vi "Get DBL.vi"(8 "error in (no error)":errorcluster, 9 "Data Type (default value)":dbl=nan, 10 "Offset":i32, 11 "JSON":string) -> (0 "error out":errorcluster, 1 "Number":dbl format="%.2f", 2 "Offset past match":i32)   [LabVIEW 2024, in "JSONtext.lvlib"]
uses:
  JSONtext.lvlib
  String Subset.vi
  Advance past Number.vi
  Parsing Error in converting to LabVIEW type.vi
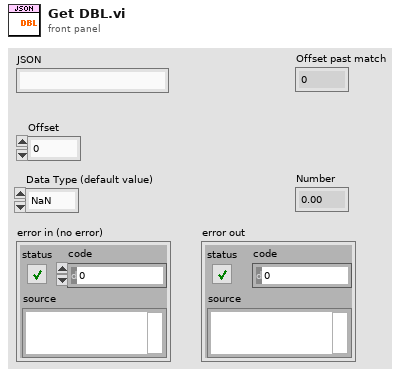
[diagram p1: front panel]
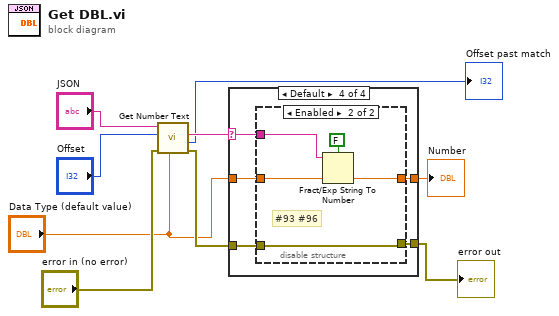
[diagram p0: block diagram]
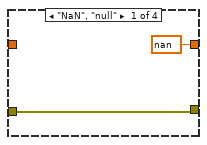
[diagram p2: hidden frame]
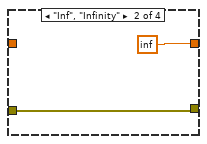
[diagram p3: hidden frame]
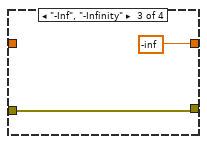
[diagram p4: hidden frame]
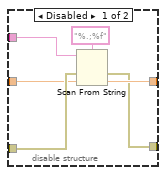
[diagram p5: hidden frame]
diagram:
  n1 = call "Get Number Text.vi"("LV Type"="Data Type (default value)", "error in (no error)"="error in (no error)", "Offset"="Offset", "JSON"="JSON") -> ("error out"=w6:errorcluster, "Offset past match"=→"Offset past match":i32, "Number Text"=w4:string)  [unwired: 4 in, 1 out]
  n2 = case shown="Default" w4 {
    selector: w4 -> [_ _ _ w16]
    tunnel: [nan ("default value 1") inf ("default value 1") -inf ("default value 1") w20] -> w3
    tunnel: w6 -> [w11 w12 w14 w19]
    tunnel: [w11 w12 w14 w18] -> w5
    tunnel: "Data Type (default value)" -> [_ _ _ w17]
    frame "NaN", "null" {
    }
    frame "Inf", "Infinity" {
    }
    frame "-Inf", "-Infinity" {
    }
    frame Default {
      n3 = disable-structure shown="Enabled" {
        disable-tunnel: [w26 w30] -> w20
        disable-tunnel: w19 -> [w25 w27]
        disable-tunnel: [w24 w27] -> w18
        disable-tunnel: w17 -> [w23 w31]
        disable-tunnel: w16 -> [w22 w29]
        frame Disabled {
          n4 = Scan From String(format string="%.;%f", input string=w22, error in=w25, default 1=w23) -> (error out=w24:errorcluster, output 1=w26:dbl)  [unwired: 1 in, 2 out]
        }
        frame Enabled {
          # "#93 #96"
          n5 = Fract/Exp String To Number(use system decimal point (T)=FALSE, string=w29, default (0 dbl)=w31) -> (number=w30:dbl)  [unwired: 1 in, 1 out]
        }
      }
    }
  }
  "error out" <- w5
  "Number" <- w3
